vi "TxPkt - Update Port Channel.vi"(8 "error in (no error)":errorcluster, 11 "Packet Ref in":T1 format="%.0x") -> (0 "error out":errorcluster, 3 "Packet Ref out":T1 format="%.0x")   [LabVIEW 2019, in "UDP-Custom-Device System Explorer.lvlib"]
uses:
  UDP-Custom-Device System Explorer.lvlib
  <vilib>/NI VeriStand/Custom Device API/Custom Device Item Ref.ctl
  <vilib>/NI VeriStand/Custom Device Tools/Custom Device Utility Library/NI VeriStand - Search for Item by Name.vi
  <vilib>/NI VeriStand/Custom Device Tools/Custom Device Utility Library/Custom Device Utility Library.lvlib
  <vilib>/NI VeriStand/Custom Device API/Custom Device API.lvlib
  Property Accessors/Tx Packet Accessors.lvlib
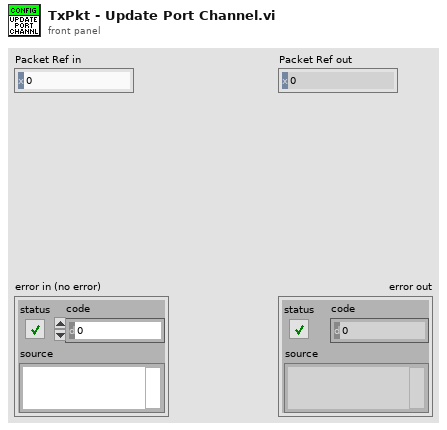
[diagram p1: front panel]
types:
  T1 = typedef "Custom Device API.lvlib/Custom Device Item Ref.ctl" = u64
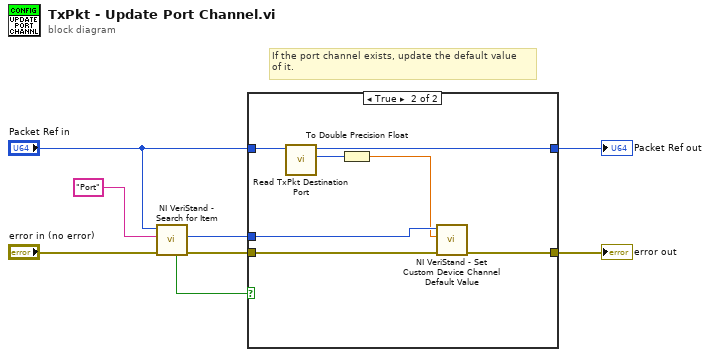
[diagram p0: block diagram]
diagram:
  # "If the port channel exists, update the default value\nof it."
  n1 = call-poly <vilib>:"NI VeriStand - Search for Item.vi"("error in"="error in (no error)", "Item Name"="Port", "Section Ref in"="Packet Ref in") -> ("error out"=w6:errorcluster, "Item Ref"=w4:T1, "Found"=w5:bool)  [unwired: 5 in, 1 out]
  n2 = case shown="True" w5 {
    tunnel: w6 -> [w9 w16]
    tunnel: w4 -> [_ w17]
    tunnel: [w10 w13] -> w3
    tunnel: "Packet Ref in" -> [w10 w14]
    tunnel: [w9 w15] -> w1
    frame False {
    }
    frame True {
      n3 = call "Read TxPkt Destination Port.vi"("Node Ptr"=w14) -> ("Destination Port"=w12:u16, "Node Ptr out"=w13:T1)  [unwired: 8 in, 1 out]
      n4 = To Double Precision Float(number=w12) -> (double precision float=w11:dbl)
      n5 = call <vilib>:"NI VeriStand - Set Custom Device Channel Default Value.vi"("error in (no error)"=w16, "Default Value"=w11, "Channel Ref in"=w17) -> ("error out"=w15:errorcluster)  [unwired: 7 in, 1 out]
    }
  }
  "error out" <- w1
  "Packet Ref out" <- w3
